vi "ROI entry-Stop trig delay blinking.vi"   [LabVIEW 2017]
uses:
  ROI Entry screen/Globals/gl_ROI Entry UI globals.vi
types:
  T1 = typedef "ROI entry screen ctrl refs cluster.ctl" = cluster{"Done button":refnum<vi>, "Imaging button":refnum<vi>, "Acquisition button":refnum<vi>, "POI dwell time (us)":refnum<vi>, "Scan dwell time per pixel (us)":refnum<vi>, "# of planes":refnum<vi>, "Zoom Ctrl":refnum<vi>, "Equal size":refnum<vi>, "Channel":refnum<vi>, "Image Display":refnum<vi>, "Z-Plane Selector":refnum<vi>, "Number of lines left":refnum<vi>, "Z-stack folder path":refnum<vi>, "POI Density":refnum<vi>, "Arb Plane Entry":refnum<vi>, "Whole plane":refnum<vi>, "Clear Last":refnum<vi>, "Clear All":refnum<vi>, "Trial Length (sec)":refnum<vi>, "Palette Type":refnum<vi>, "Intensity slider":refnum<vi>, "# POI":refnum<vi>, "Max Z Proj":refnum<vi>, "Zplane ind":refnum<vi>, "Wavelength (nm)":refnum<vi>, "Number of Trials":refnum<vi>, "Funct stim.trig.enable":refnum<vi>, "Funct stim.trig.delay (s)":refnum<vi>, "Line Mode":refnum<vi>, "Step size (µm)":refnum<vi>, "ROI move mode":refnum<vi>, "Cool-down time (s)":refnum<vi>, "Enable cool-down time":refnum<vi>, "Motor Z ind. (um)":refnum<vi>, "AOL Z ind. (um)":refnum<vi>, "Load Reference Image":refnum<vi>}
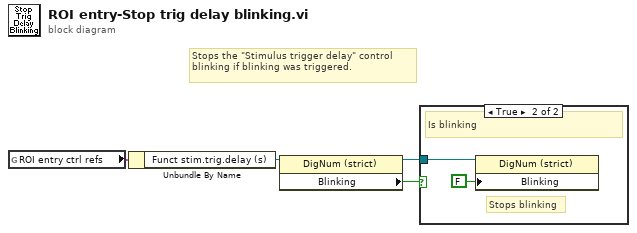
[diagram p0: block diagram]
diagram:
  # "Stops the \"Stimulus trigger delay\" control blinking if blinking was triggered."
  n1 = global read "gl_ROI Entry UI globals.vi" "ROI entry ctrl refs"() -> (w1:T1)
  n2 = Unbundle By Name(w1) -> ("Funct stim.trig.delay (s)"=w2:refnum<vi>)
  n3 = property on="Property Node" class="DigNum (strict)"(reference=w2) -> (reference out=w4:refnum<vi>, "Blinking"=w3:bool)  [unwired: 1 in, 1 out]
  n4 = case shown="True" w3 {
    tunnel: w4 -> [_ w5]
    frame False {
    }
    frame True {
      # "Stops blinking"
      # "Is blinking"
      n5 = property on="Property Node" class="DigNum (strict)"(reference=w5, "Blinking"=FALSE) -> ()  [unwired: 1 in, 2 out]
    }
  }
